vi "KG get temp lcl.vi"(8 "Fehler (Eingang, kein Fehler)":errorcluster, 10 "controller":u32, 11 "VISA-Ressourcenname":refnum<visa-resource-name>) -> (0 "Fehler (Ausgang)":errorcluster, 1 "Kommando gesendet":string, 2 "temp":dbl, 3 "VISA-Ressourcenname (Ausgang)":refnum<visa-resource-name>)   [LabVIEW 2020, in "Linearisierung v2.lvlib" / "Gasteiler.lvlib" / "HovaCAL_Interface.lvlib" / "KGN.lvlib" / "get.lvlib"]
uses:
  get.lvlib
  KGN.lvlib
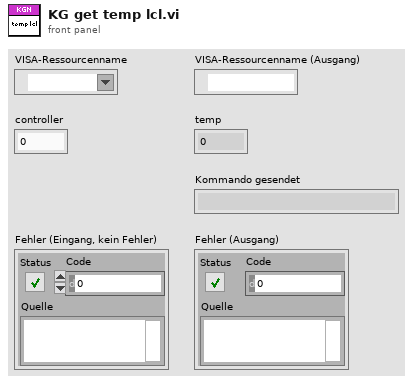
[diagram p1: front panel]
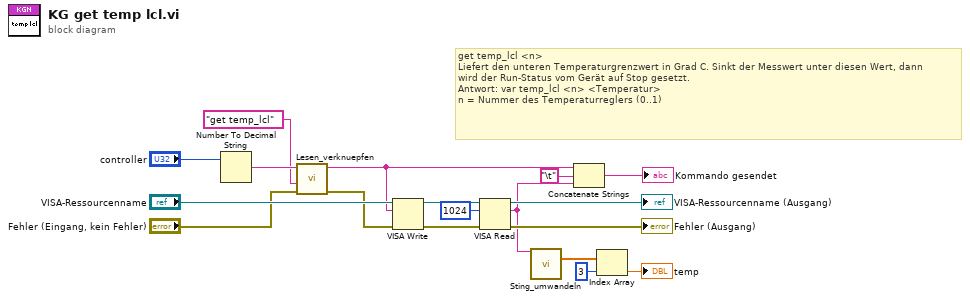
[diagram p0: block diagram]
diagram:
  # "get temp_lcl <n>\nLiefert den unteren Temperaturgrenzwert in Grad C. Sinkt der Messwert unter diesen Wert, dann\nwird der Run-Status vom Gerät auf Stop gesetzt.\nAntwort: var temp_lcl <n> <Temperatur>\nn = Nummer des Temperaturreglers (0..1)"
  n1 = Number To Decimal String(number="controller") -> (decimal integer string=w8:string)  [unwired: 1 in]
  n2 = call "Lesen_verknuepfen.vi"("error in (no error)"="Fehler (Eingang, kein Fehler)", "Order"="get temp_lcl" ("Schreibpuffer"), "param"=w8) -> ("error out"=w10:errorcluster, "Verknüpfter String"=w9:string)  [unwired: 7 in]
  n3 = VISA Write(VISA resource name="VISA-Ressourcenname", write buffer=w9, error in (no error)=w10) -> (VISA resource name out=w18:refnum<visa-resource-name>, error out=w17:errorcluster)  [unwired: 1 out]
  n4 = VISA Read(VISA resource name=w18, byte count=u32 1024 ("Byte-Anzahl"), error in (no error)=w17) -> (VISA resource name out=→"VISA-Ressourcenname (Ausgang)":refnum<visa-resource-name>, read buffer=w2:string, error out=→"Fehler (Ausgang)":errorcluster)  [unwired: 1 out]
  n5 = call "Sting_umwandeln.vi"("Lesepuffer"=w2) -> ("Zahl array"=w5:dbl[])  [unwired: 8 in, 6 out]
  n6 = Concatenate Strings(w9, "\t", w2) -> (→"Kommando gesendet":string)
  n7 = Index Array(array=w5, index=3 ("Index")) -> (element=→"temp":dbl)
